vi "launch labview if not running.vi"(8 "error in":errorcluster, 11 "desired lv version":dbl) -> (0 "error out":errorcluster, 1 "newly opened":bool, 2 "port":u32, 3 "vi server available":bool, 5 "labview directory":path)   [LabVIEW 2013]
uses:
  <vilib>/Utility/config.llb/Read Key (String).vi
  <vilib>/Utility/config.llb/Read Key (U32).vi
  <vilib>/Utility/config.llb/NI_LVConfig.lvlib
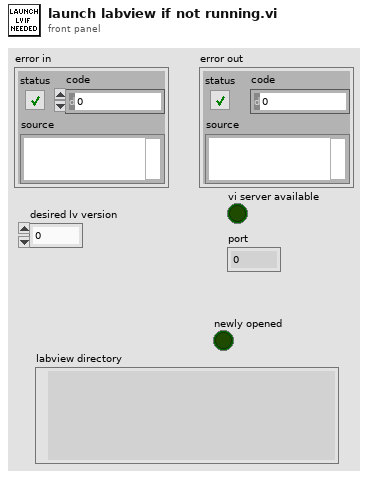
[diagram p1: front panel]
types:
  T1 = typedef "NI_LVConfig.lvlib/Config Data RefNum.ctl" = refnum<k1>
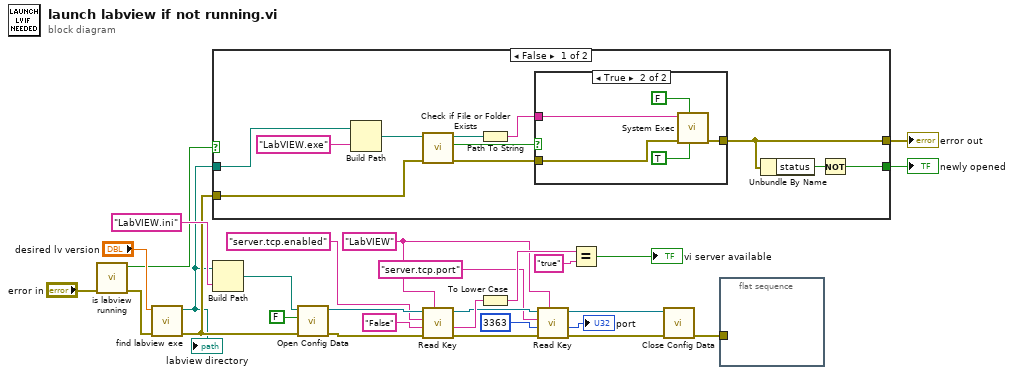
[diagram p0: block diagram]
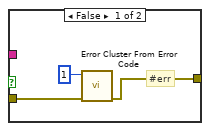
[diagram p2: hidden frame]
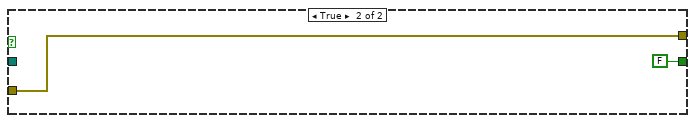
[diagram p3: hidden frame]
diagram:
  w4 = "LabVIEW" ("section")
  n1 = call "is labview running.vi"("error in"="error in") -> ("error out"=w27:errorcluster, "running"=w18:bool)  [unwired: 9 in]
  n2 = call "find labview exe.vi"("error in"=w27, "desired lv version"="desired lv version") -> ("error out"=w16:errorcluster, "labview directory"=w14:path)  [unwired: 8 in]
  "labview directory" <- w14
  n3 = case shown="False" w18 {
    tunnel: [w32 w49] -> w17
    tunnel: w16 -> [w30 w49]
    tunnel: [w31 FALSE] -> w15
    tunnel: w14 -> [w29 _]
    frame False {
      n4 = Build Path(base path=w29, name or relative path="LabVIEW.exe") -> (appended path=w33:path)
      n5 = call <vilib>:"Check if File or Folder Exists.vi"("error in (no error)"=w30, "path"=w33) -> ("error out"=w38:errorcluster, "file or folder exists?"=w39:bool, "dup path"=w37:path)  [unwired: 7 in]
      n6 = Path To String(path=w37) -> (string=w36:string)
      n7 = case shown="True" w39 {
        tunnel: [w41 w46] -> w32
        tunnel: w38 -> [w42 w47]
        tunnel: w36 -> [_ w45]
        frame False {
          # "#err"
          n8 = call <vilib>:"Error Cluster From Error Code.vi"("error in (no error)"=w42, "error code (0)"=1) -> ("error out"=w41:errorcluster)  [unwired: 7 in]
        }
        frame True {
          n9 = call <vilib>:"System Exec.vi"("run minimized? (F)"=TRUE, "wait until completion? (T)"=FALSE, "error in (no error)"=w47, "command line"=w45) -> ("error out"=w46:errorcluster)  [unwired: 4 in, 3 out]
        }
      }
      n10 = Unbundle By Name(w32) -> ("status"=w35:bool)
      n11 = Not(x=w35) -> (.not. x?=w31:bool)
    }
    frame True {
    }
  }
  "error out" <- w17
  "newly opened" <- w15
  n12 = Build Path(base path=w14, name or relative path="LabVIEW.ini") -> (appended path=w20:path)
  n13 = call <vilib>:"Open Config Data.vi"("error in (no error)"=w16, "create file if necessary (T)"=FALSE, "configuration file path"=w20) -> ("error out"=w8:errorcluster, "refnum"=w9:T1)  [unwired: 6 in, 1 out]
  n14 = call-poly <vilib>:"Read Key.vi"("section"=w4, "error in (no error)"=w8, "default value"="False", "key"="server.tcp.enabled", "refnum"=w9) -> ("error out"=w10:errorcluster, "value"=w19:string, "refnum out"=w11:T1)  [unwired: 3 in, 1 out]
  n15 = To Lower Case(string=w19) -> (all lower case string=w23:string)
  n16 = call-poly <vilib>:"Read Key.vi"("section"=w4, "error in (no error)"=w10, "default value"=u32 3363, "key"="server.tcp.port", "refnum"=w11) -> ("error out"=w13:errorcluster, "value"=→"port":u32, "refnum out"=w12:T1)  [unwired: 3 in, 1 out]
  n17 = Equal?(x=w23, y="true") -> (x = y?=→"vi server available":bool)
  n18 = call <vilib>:"Close Config Data.vi"("error in (no error)"=w13, "refnum"=w12) -> ("error out"=w1:errorcluster)  [unwired: 8 in, 1 out]
  n19 = flat-sequence {
    tunnel: w1 -> [_]
    frame #0 {
    }
  }
